vi "get_mass.vi"(11 "Data In":string) -> (3 "Data Out":string)   [LabVIEW 2018, in "Labview Python.lvlib"]
uses:
  Labview Python.lvlib
  Post Analysis/Post Analysis.lvlib
panel:
  out "Statistics":T1
  out "Certainty of First Q State":T2(graph)
  out "Freq and Mass vs Time":cluster{"Scan #":dbl[], dbl[]}[](graph)
  out "JSON string":string
  in  "output cluster":T3
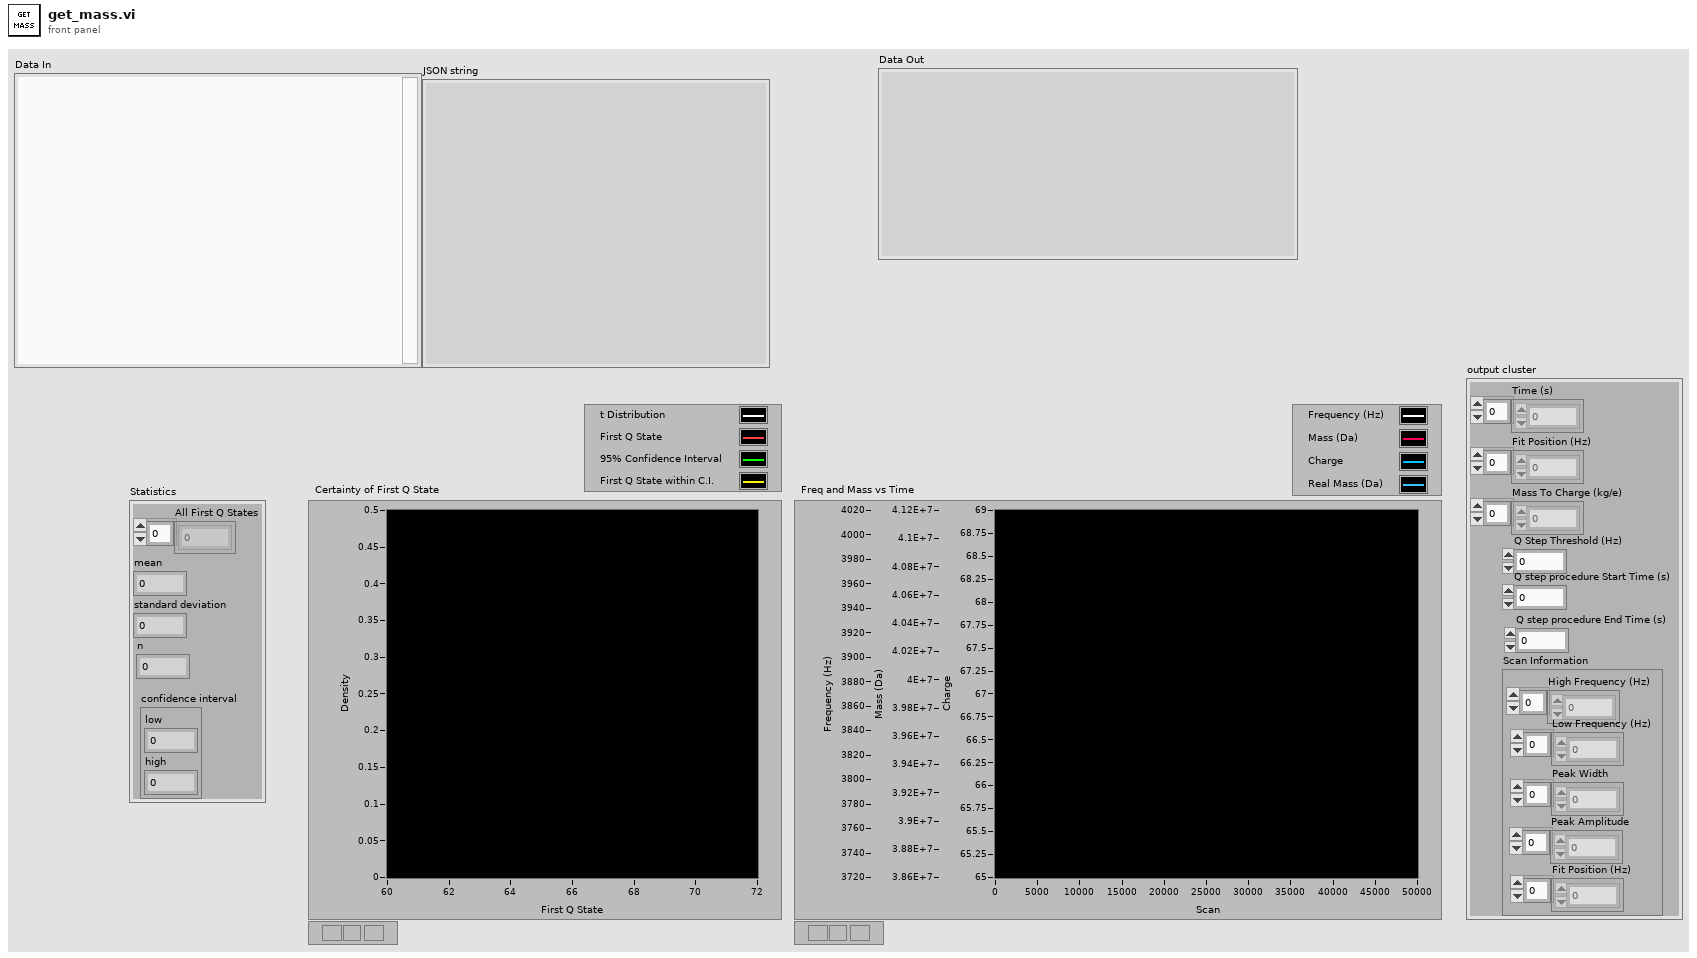
[diagram p1: front panel]
types:
  T1 = cluster{"All First Q States":dbl[], "mean":dbl, "standard deviation":dbl, "n":i32, "confidence interval":cluster{"low":dbl, "high":dbl}}
  T2 = cluster{"Ramp Pattern":dbl[], "All First Q States":dbl[]}[]
  T3 = cluster{"Time (s)":dbl[], "Fit Position (Hz)":dbl[], "Mass To Charge (kg/e)":dbl[], "Q Step Threshold (Hz)":dbl, "Q step procedure Start Time (s)":dbl, "Q step procedure End Time (s)":dbl, "Scan Information":cluster{"High Frequency (Hz)":dbl[], "Low Frequency (Hz)":dbl[], "Peak Width":dbl[], "Peak Amplitude":dbl[], "Fit Position (Hz)":dbl[]}}
  T4 = cluster{"High Frequency (Hz)":dbl[], "Peak Width":dbl[], "Peak Amplitude":dbl[], "Low Frequency (Hz)":dbl[], "Fit Position (Hz)":dbl[]}
  T5 = cluster{"High Frequency (Hz)":dbl[], "Low Frequency (Hz)":dbl[], "Peak Width":dbl[], "Peak Amplitude":dbl[], "Fit Position (Hz)":dbl[]}
  T6 = typedef "Post Analysis.lvlib/Mass Calc Output.ctl" = cluster{"Time (s)":dbl[], "Mass (kg)":dbl[], "Charge (e)":dbl[], "Mass/Charge (kg/e)":dbl[]}
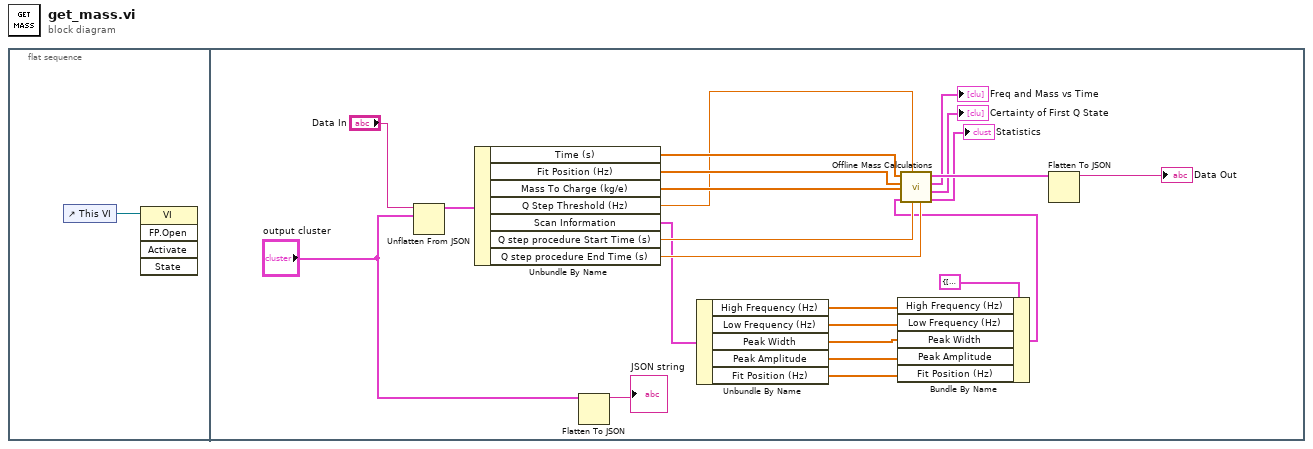
[diagram p0: block diagram]
diagram:
  n1 = flat-sequence {
    frame #0 {
      n2 = control-ref of="This VI"() -> (w1:refnum<vi>)
      n3 = invoke class="VI" method="FP.Open"(reference=w1) -> ()  [unwired: 4 in, 5 out]
    }
    frame #1 {
      n4 = Unflatten From JSON(JSON string="Data In", type and defaults="output cluster") -> (value=w24:T3)  [unwired: 5 in, 1 out]
      n5 = Unbundle By Name(w24) -> ("Time (s)"=w23:dbl[], "Fit Position (Hz)"=w22:dbl[], "Mass To Charge (kg/e)"=w21:dbl[], "Q Step Threshold (Hz)"=w20:dbl, "Scan Information"=w12:T5, "Q step procedure Start Time (s)"=w19:dbl, "Q step procedure End Time (s)"=w18:dbl)
      n6 = Flatten To JSON(anything="output cluster") -> (JSON string=→"JSON string":string)  [unwired: 2 in, 1 out]
      n7 = Unbundle By Name(w12) -> ("High Frequency (Hz)"=w11:dbl[], "Low Frequency (Hz)"=w10:dbl[], "Peak Width"=w9:dbl[], "Peak Amplitude"=w8:dbl[], "Fit Position (Hz)"=w7:dbl[])
      n8 = Bundle By Name(cluster=T4 {"High Frequency (Hz)"=[], "Peak Width"=[], "Peak Amplitude"=[], "Low Frequency (Hz)"=[], "Fit Position (Hz)"=[]} ("Scan Information"), "High Frequency (Hz)"=w11, "Low Frequency (Hz)"=w10, "Peak Width"=w9, "Peak Amplitude"=w8, "Fit Position (Hz)"=w7) -> (w6:T4)
      n9 = call "Offline Mass Calculations.vi"("Q step procedure End Time (s)"=w18, "Q step procedure Start Time (s)"=w19, "Q Step Threshold (Hz)"=w20, "Scan Information"=w6, "Mass To Charge (kg/e)"=w21, "Fit Position (Hz)"=w22, "Time (s)"=w23) -> ("Statistics"=→"Statistics":T1, "Certainty of First Q State"=→"Certainty of First Q State":T2, "Freq and Mass vs Time"=→"Freq and Mass vs Time":cluster{"Scan #":dbl[], dbl[]}[], "Data Out"=w5:T6)  [unwired: 1 in]
      n10 = Flatten To JSON(anything=w5) -> (JSON string=→"Data Out":string)  [unwired: 2 in, 1 out]
    }
  }
